vi "Configure Integration Timer.vi"(5 "Element (0:ALL)":i32(ring) items=["All", "1", "2", "3", "4", "5", "6"], 7 "Hour (00000 h)":i32 min=0 max=10000 step=1 format="%05.0f", 8 "error in (no error)":errorcluster, 9 "Second (00 s)":i32 min=0 max=59 format="%02.0f", 10 "Minute (00 m)":i32 min=0 max=59 step=1 format="%02.0f", 11 "VISA resource name":refnum<visa-resource-name>) -> (0 "error out":errorcluster, 3 "VISA resource name out":refnum<visa-resource-name>)   [LabVIEW 2021, in "Yokogawa WT1800 Series.lvlib"]
doc: "Configures the integration timer features."
uses:
  <instrlib>/Yokogawa WT1800 Series/Yokogawa WT1800 Series.lvlib
panel:
  # "h"
  # "m"
  # "s"
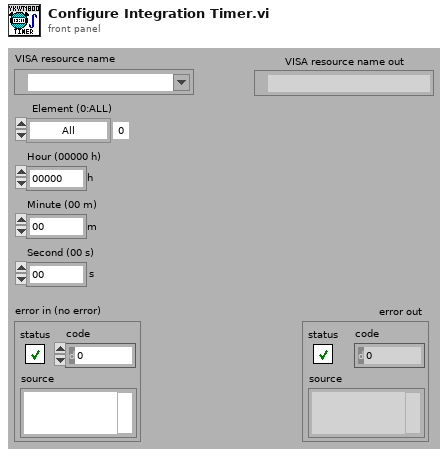
[diagram p1: front panel]
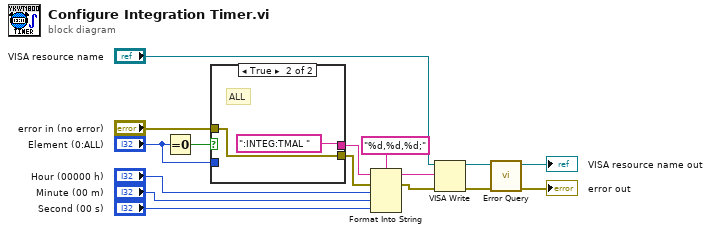
[diagram p0: block diagram]
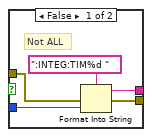
[diagram p2: hidden frame]
diagram:
  n1 = Equal To 0?(x="Element (0:ALL)") -> (x = 0?=w10:bool)
  n2 = case shown="True" w10 {
    tunnel: "error in (no error)" -> [w20 w23]
    tunnel: [w19 w23] -> w5
    tunnel: [w18 ":INTEG:TMAL "] -> w4
    tunnel: "Element (0:ALL)" -> [w17 _]
    frame False {
      # "Not ALL"
      n3 = Format Into String ("文字列にフォーマット")(format string=":INTEG:TIM%d " ("形式文字列"), error in=w20, w17) -> (resulting string=w18:string, error out=w19:errorcluster)  [unwired: 1 in]
    }
    frame True {
      # "ALL"
    }
  }
  n4 = Format Into String ("文字列にフォーマット")(format string="%d,%d,%d;" ("形式文字列"), initial string=w4, error in=w5, "Hour (00000 h)", "Minute (00 m)", "Second (00 s)") -> (resulting string=w3:string, error out=w2:errorcluster)
  n5 = VISA Write ("VISA書き込み")(VISA resource name="VISA resource name", write buffer=w3, error in (no error)=w2) -> (VISA resource name out=w16:refnum<visa-resource-name>, error out=w15:errorcluster)  [unwired: 1 out]
  n6 = call <instrlib>:"Error Query.vi"("error in (no error)"=w15, "VISA resource name"=w16) -> ("error out"=→"error out":errorcluster, "VISA resource name out"=→"VISA resource name out":refnum<visa-resource-name>)  [unwired: 6 in, 2 out]
